vi "SetUpN1911a.vi"(2 "error in (no error)":errorcluster) -> (0 "error out":errorcluster)   [LabVIEW 2009]
doc: "Set up defaults for N1911A average power measurements which disable automatic parameter selection. \nThese are the modes used most frequently to measure power from the signal generator or noise generato"
panel:
  in  "SCPI commands":string="*cls\nSYST:PRES DEF\nSENS:FREQ 2850MHz\nSENS:AVER:SDET OFF\nSENS:MRAT DOUBLE\nSENS:BAND:VID OFF\nSENS:AVER:COUNT 2\nSENS:AVER:COUNT:AUTO OFF\nSENS:AVER:STATE ON\nDISP:WIND1:FORM DNUM\ncalc1:feed1 \"pow:aver\"\ncalc3:feed1 \"pow:ptav\"\nDISP:WIND1:NUM1:RES 4\nDISP:WIND1:NUM2:RES 4\nSYST:REM\n"
  # "Set up defaults for N1911A average power measurements for stationary signals such\nas CW from a signal generator or white noise from a noise generator.\nThese are the modes used most frequently to measure power from generators that are not triggered sources.  For pulsed transmitters, use different defaults expressed as a different list of SCPI commands.\nFrequency setting seems to be good for entire S-Band"
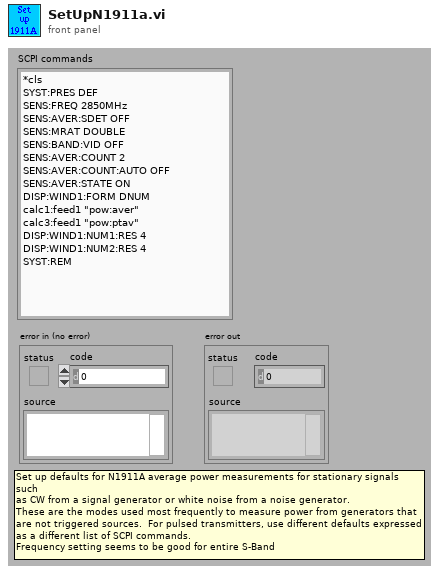
[diagram p1: front panel]
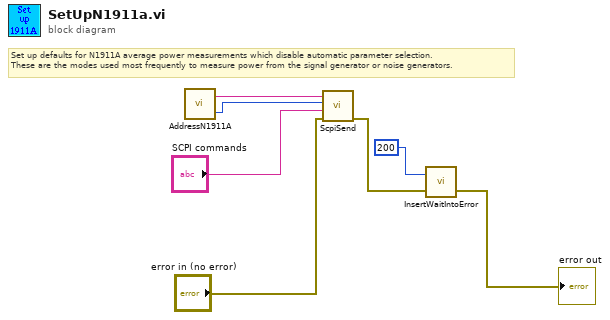
[diagram p0: block diagram]
diagram:
  # "Set up defaults for N1911A average power measurements which disable automatic parameter selection. \nThese are the modes used most frequently to measure power from the signal generator or noise generators."
  n1 = call "AddressN1911A.vi"() -> ("Port"=w5:i32, "IP address"=w6:string)  [unwired: 2 in]
  n2 = call "ScpiSend.vi"("error in (no error)"="error in (no error)", "Command"="SCPI commands", "TCP port"=w5, "IP Address"=w6) -> ("error out"=w3:errorcluster)  [unwired: 7 in]
  n3 = call "InsertWaitIntoError.vi"("error in (no error)"=w3, "Wait (msecs)"=200 ("PauseBeforeFirstReading")) -> ("error out"=→"error out":errorcluster)  [unwired: 1 in]
